vi "禹山浊度_获取温度和测量值.vi"(8 "error in (no error)":errorcluster caption="错误输入（无错误）", 11 "MB session in":refnum<class "MB_Master.lvclass">) -> (0 "error out":errorcluster caption="错误输出", 2 "输出值":cluster{"温度测量值":sgl, "浊度":sgl}, 3 "MB session out":refnum<class "MB_Master.lvclass">)   [LabVIEW 2022 SP3, in "斯坦道多参数.lvlib"]
uses:
  <vilib>/Plasmionique/MB Master/MB_Master/MB_Master.lvclass
  <vilib>/Plasmionique/MB Master/MB Master.lvlib
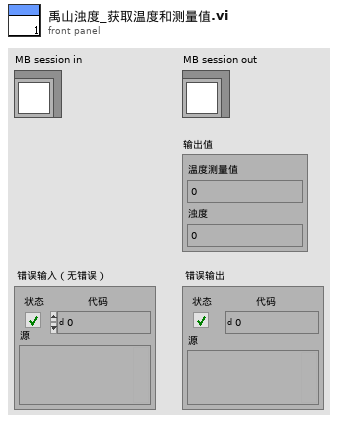
[diagram p1: front panel]
types:
  T1 = cluster{"pH":u32, "DO":u32, "Cond":u32, "Turb":u32, "叶绿素a":u32, "藻密度":u32, "ORP":u32, "COD":u32, "氯化物":u32, "氨氮":u32, "水中油":u32, "悬浮物":u32, "余氯":u32}
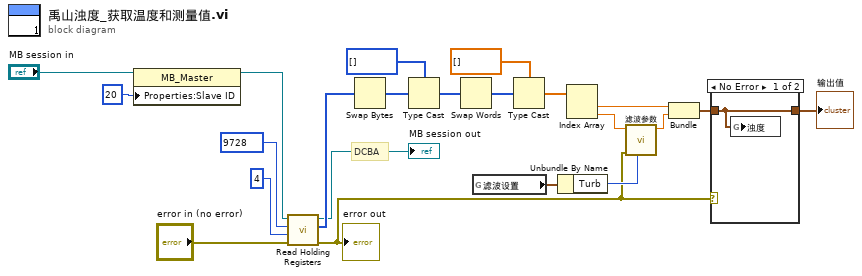
[diagram p0: block diagram]
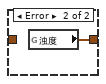
[diagram p2: hidden frame]
diagram:
  # "DCBA"
  n1 = property class="MB_Master"(reference="MB session in", "Properties:Slave ID"=u16 20 ("y")) -> (reference out=w14:refnum<class "MB_Master.lvclass">)  [unwired: 1 in, 1 out]
  n2 = call <vilib>:"Read Holding Registers.vi"("error in (no error)"="error in (no error)", "quantity"=u16 4, "starting address"=u16 9728, "MB session in"=w14) -> ("error out"=w1:errorcluster, "Registers"=w12:u16[], "MB session out"=→"MB session out":refnum<class "MB_Master.lvclass">)  [unwired: 5 in]
  "error out" <- w1
  n3 = Swap Bytes(anything=w12) -> (byte swapped=w11:u16[])
  n4 = Type Cast(type=u32[] [] ("数组 2"), x=w11) -> (*(type *) &x=w18:u32[])
  n5 = Swap Words(1:w18) -> (0:w20:u32[])
  n6 = global read "断电保存变量.vi" "滤波设置"() -> (w4:T1)
  n7 = Type Cast(type=sgl[] [] ("数组 2"), x=w20) -> (*(type *) &x=w16:sgl[])
  n8 = Unbundle By Name(w4) -> ("Turb"=w3:u32)
  n9 = Index Array(array=w16) -> (element #1=w10:sgl, element #2=w6:sgl)  [unwired: 2 in]
  n10 = call "滤波参数.vi"("滤波次数"=w3, "error in (no error)"=w1, "x"=w6) -> ("mode"=w5:dbl)  [unwired: 7 in, 1 out]
  n11 = Bundle("数值"=w10, "mode"=w5) -> (w9:cluster{"数值":sgl, "mode":dbl})  [unwired: 1 in]
  n12 = case shown="No Error" w1 {
    tunnel: w9 -> [w23 _]
    tunnel: [w23 w24] -> w2
    frame No Error {
      n13 = global write "禹山过程全局变量.vi" "浊度"(w23) -> ()
    }
    frame Error {
      n14 = global read "禹山过程全局变量.vi" "浊度"() -> (w24:cluster{"温度测量值":sgl, "浊度测量值":sgl})
    }
  }
  "输出值" <- w2
